vi "Control - Generic - Wastegate Host.vi"() -> ()   [LabVIEW 2015, in "ECS-Host.lvlib"]
uses:
  ECS-Host.lvlib
panel:
  in  "WgPsn_PIDE":bool caption="ManualWGSetpointEnable"
  out "MAPStp":sgl caption="[kPa]"
  out "MAP":sgl caption="[kPa]"
  in  "WgPsn_Max":sgl caption="[%Open]"
  in  "WgPsn_Min":sgl caption="[%Open]"
  in  "WgPsn_PIDMax":sgl caption="[V]"
  in  "WgPsn_PIDMin":sgl caption="[V]"
  in  "WgPsn_Kp":sgl caption="[V]"
  in  "WgPsn_Ti":sgl caption="[V]"
  in  "WgPsn_Td":sgl caption="[V]"
  out "WgPsn_Des":sgl caption="[%Open]"
  out "WgPsn_PIDOut":sgl caption="[V]"
  in  "WgPsn_ManE":bool caption="ManualWGSetpointEnable"
  in  "WgPsn_Man":sgl caption="[%Open]"
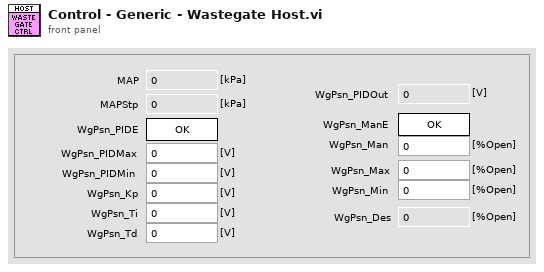
[diagram p1: front panel]
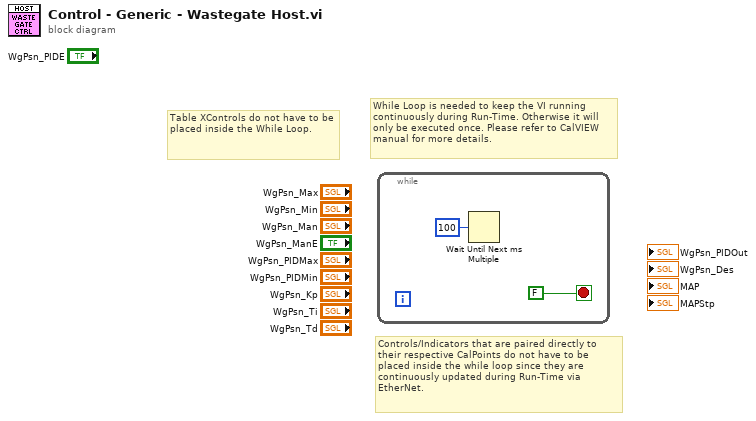
[diagram p0: block diagram]
diagram:
  # "Table XControls do not have to be placed inside the While Loop."
  # "While Loop is needed to keep the VI running\ncontinuously during Run-Time. Otherwise it will only be executed once. Please refer to CalVIEW manual for more details."
  # "Controls/Indicators that are paired directly to their respective CalPoints do not have to be placed inside the while loop since they are continuously updated during Run-Time via EtherNet."
  n1 = while {
    stop <- FALSE stop-if-true
    n2 = Wait Until Next ms Multiple(millisecond multiple=u32 100) -> ()  [unwired: 1 out]
  }
